vi "Pre Launch Init.vi"(11 "TranslationStageUI.lvclass":refnum<class "TranslationStageUI.lvclass">) -> (0 "error out":errorcluster, 3 "TranslationStageUI.lvclass":refnum<class "TranslationStageUI.lvclass">)   [LabVIEW 2023, in "TranslationStage Library.lvlib" / "TranslationStage_UI.lvlib" / "TranslationStageUI.lvclass"]
doc: "(<B>Filename</B>: Actor Framework.lvlib:Actor.lvclass:Pre Launch Init.vi)\n\nDefines behavior that occurs after the Launch Nested Actor method is invoked but before the actor's Actor Core method begins running.\n\nBy default, this method does nothing. A descendant class may override it to define behavior."
uses:
  TranslationStageUI.lvclass
  StageMoveDone_For_UI.ctl
  TranslationStageUI.lvclass/TranslationStageUI.ctl
  <vilib>/ActorFramework/Actor/Actor.lvclass
  typedefs/typedefs.lvlib
panel:
  in  "Variant":variant
  in  "Registers":u16[][](array[numeric])
  in  "Positions":T1={"CH1 Pos"=0.0, "CH2 Pos"=0.0, "CH3 Pos"=0.0, "CH4 Pos"=0.0, "Home?"=TRUE}
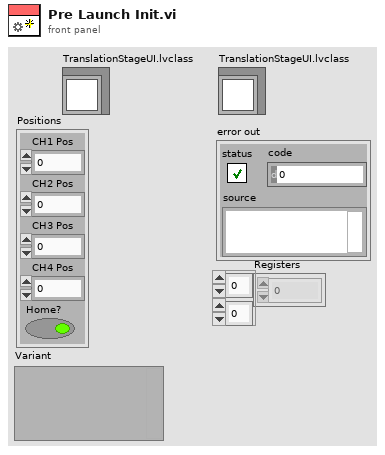
[diagram p1: front panel]
types:
  T1 = typedef "typedefs.lvlib/StageMoveDone_For_UI.ctl" = cluster{"CH1 Pos":sgl, "CH2 Pos":dbl, "CH3 Pos":dbl, "CH4 Pos":dbl, "Home?":bool}
  T2 = cluster{"Scanning Done":bool, "Axis":enum16{"X", "Y", "Z", "HOM"}}
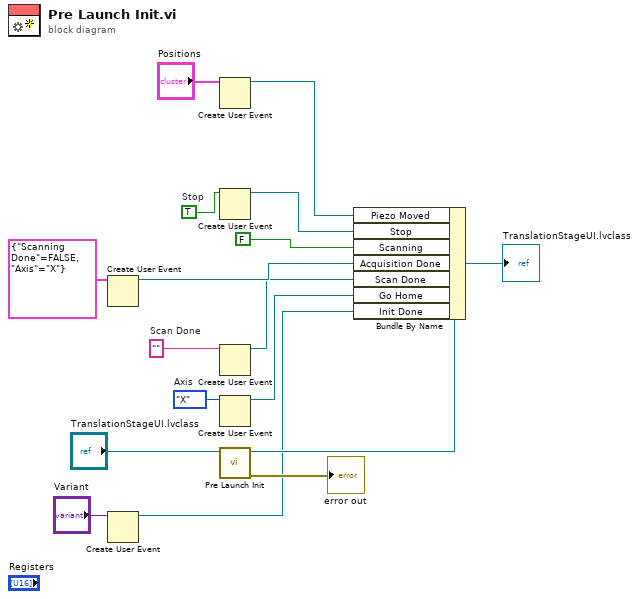
[diagram p0: block diagram]
diagram:
  w3 = enum16{"X", "Y", "Z", "HOM"}."X"  # Axis
  w9 = ""  # Scan Done
  w15 = TRUE  # Stop
  n1 = Create User Event(user event datatype=T2 {"Scanning Done"=FALSE, "Axis"=enum."X"} ("Acq Done Data")) -> (user event=w10:refnum<user-event>)  [unwired: 1 in, 1 out]
  n2 = Create User Event(user event datatype="Variant") -> (user event=w1:refnum<user-event>)  [unwired: 1 in, 1 out]
  n3 = Create User Event(user event datatype="Positions") -> (user event=w7:refnum<user-event>)  [unwired: 1 in, 1 out]
  n4 = Create User Event(user event datatype=w15) -> (user event=w16:refnum<user-event>)  [unwired: 1 in, 1 out]
  n5 = Create User Event(user event datatype=w9) -> (user event=w8:refnum<user-event>)  [unwired: 1 in, 1 out]
  n6 = Create User Event(user event datatype=w3) -> (user event=w4:refnum<user-event>)  [unwired: 1 in, 1 out]
  n7 = call-parent "Pre Launch Init.vi"("Actor in"="TranslationStageUI.lvclass") -> ("error out"=→"error out":errorcluster, "Actor out"=w11:refnum<class "TranslationStageUI.lvclass">)  [unwired: 9 in]
  n8 = Bundle By Name(cluster=w11, "Piezo Moved"=w7, "Stop"=w16, "Scanning"=FALSE ("Cam Connected"), "Acquisition Done"=w10, "Scan Done"=w8, "Go Home"=w4, "Init Done"=w1) -> (→"TranslationStageUI.lvclass":refnum<class "TranslationStageUI.lvclass">)
